vi "IACtrl_v2.vi"(7 "Irrigate?":bool=TRUE, 8 "Max Limit [mmHg]":dbl, 9 "E-Stop Vacuum":bool=TRUE, 10 "Vacuum Force [mmHg]":dbl) -> (1 "Accurus ChB Vout":dbl, 2 "Accurus ChA Vout":dbl, 3 "Accurus Engaged Vout":dbl, 6 "Vac Disp [mmHg]":i32)   [LabVIEW 2016]
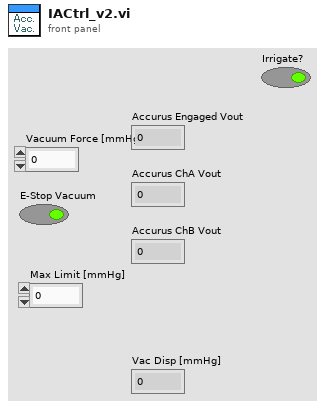
[diagram p1: front panel]
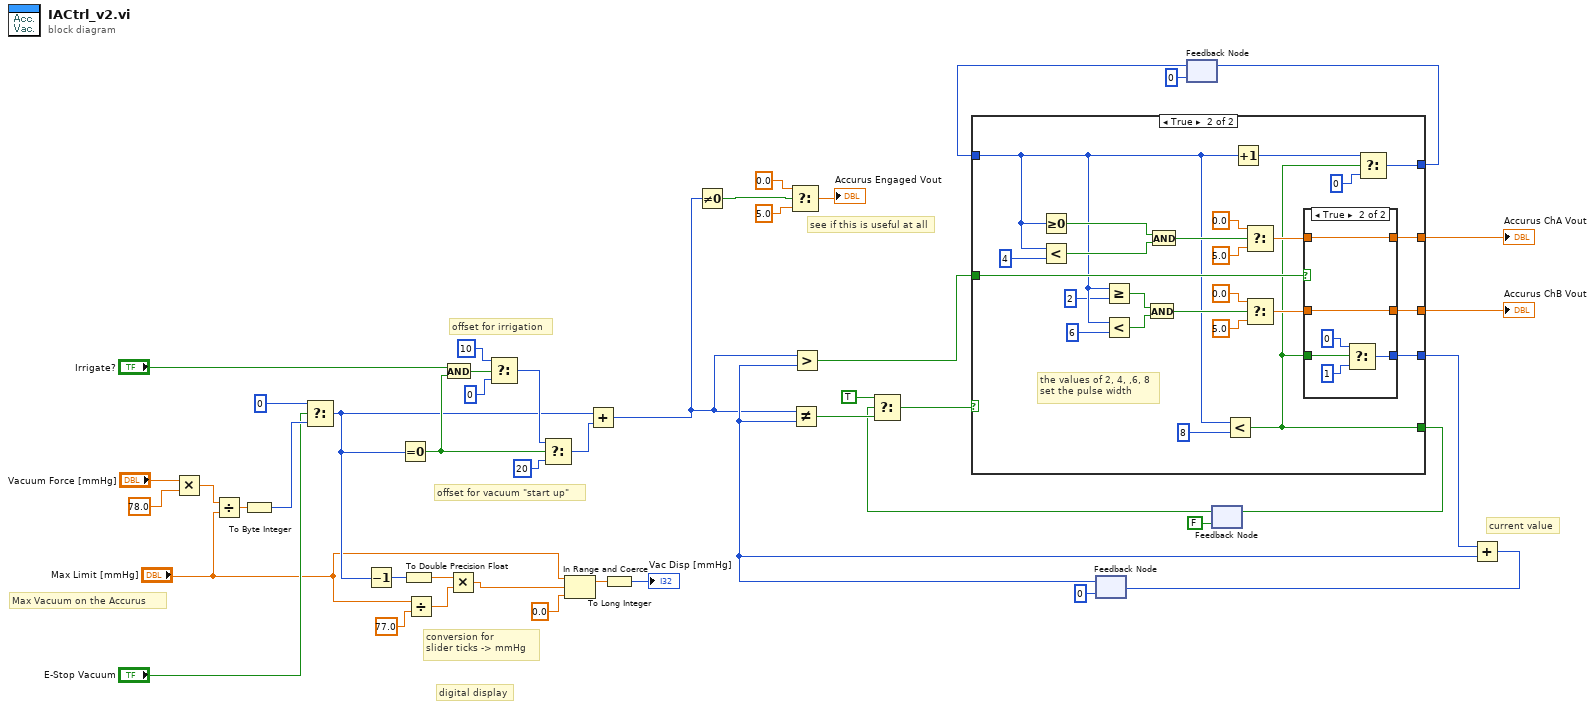
[diagram p0: block diagram]
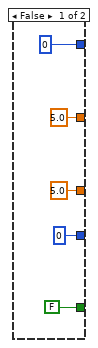
[diagram p2: hidden frame]
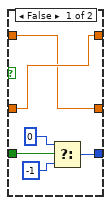
[diagram p3: hidden frame]
diagram:
  # "see if this is useful at all"
  # "digital display"
  # "offset for irrigation"
  # "Max Vacuum on the Accurus"
  # "conversion for\nslider ticks -> mmHg"
  # "offset for vacuum \"start up\""
  # "current value"
  n1 = Multiply(x="Vacuum Force [mmHg]", y=78.0) -> (x*y=w2:dbl)
  n2 = Divide(x=w2, y="Max Limit [mmHg]") -> (x/y=w16:dbl)
  n3 = To Byte Integer(number=w16) -> (8bit integer=w8:i8)
  n4 = Select(t=i8 0, s="E-Stop Vacuum", f=w8) -> (s? t:f=w7:i8)
  n5 = Decrement(x=w7) -> (x-1=w20:i8)
  n6 = Equal To 0?(x=w7) -> (x = 0?=w15:bool)
  n7 = To Double Precision Float(number=w20) -> (double precision float=w46:dbl)
  n8 = Divide(x="Max Limit [mmHg]", y=77.0) -> (x/y=w18:dbl)
  n9 = And(x="Irrigate?", y=w15) -> (x .and. y?=w14:bool)
  n10 = Multiply(x=w46, y=w18) -> (x*y=w17:dbl)
  n11 = Select(t=i8 10, s=w14, f=i8 0 ("t")) -> (s? t:f=w10:i8)
  n12 = Select(t=w10, s=w15, f=i8 20) -> (s? t:f=w43:i8)
  n13 = In Range and Coerce(upper limit="Max Limit [mmHg]", x=w17, lower limit=0.0) -> (coerced(x)=w21:dbl)  [unwired: 1 out]
  n14 = Add(x=w7, y=w43) -> (x+y=w9:i8)
  n15 = To Long Integer(number=w21) -> (32bit integer=→"Vac Disp [mmHg]":i32)
  n16 = Not Equal To 0?(x=w9) -> (x != 0?=w11:bool)
  n17 = Select(t=0.0, s=w11, f=5.0) -> (s? t:f=→"Accurus Engaged Vout":dbl)
  n18 = feedback #1(i8 0) -> (w29:i8)
  n19 = Not Equal?(x=w9, y=w29) -> (x != y?=w35:bool)
  n20 = Greater?(x=w9, y=w29) -> (0:w25:bool)
  n21 = feedback #2(i8 0) -> (w31:i8)
  n22 = feedback #3(FALSE) -> (w32:bool)
  n23 = Select(t=TRUE, s=w32, f=w35) -> (s? t:f=w34:bool)
  n24 = case shown="True" w34 {
    tunnel: [5.0 ("f") w64] -> w39
    tunnel: [5.0 ("f") w63] -> w40
    tunnel: [i8 0 ("f") w61] -> w28
    tunnel: [FALSE w56] -> w24
    tunnel: w25 -> [_ w62]
    tunnel: [i8 0 w58] -> w26
    tunnel: w31 -> [_ w60]
    frame False {
    }
    frame True {
      # "the values of 2, 4, ,6, 8 \nset the pulse width"
      n25 = Greater Or Equal To 0?(x=w60) -> (x >= 0?=w71:bool)
      n26 = Less?(x=w60, y=i8 4) -> (x < y?=w70:bool)
      n27 = Greater Or Equal?(x=w60, y=i8 2) -> (x >= y?=w69:bool)
      n28 = Less?(x=w60, y=i8 6) -> (x < y?=w68:bool)
      n29 = And(x=w69, y=w68) -> (x .and. y?=w67:bool)
      n30 = And(x=w71, y=w70) -> (x .and. y?=w72:bool)
      n31 = Less?(x=w60, y=i8 8) -> (x < y?=w56:bool)
      n32 = Increment(x=w60) -> (x+1=w59:i8)
      n33 = Select(t=0.0, s=w72, f=5.0) -> (s? t:f=w66:dbl)
      n34 = Select(t=0.0, s=w67, f=5.0) -> (s? t:f=w65:dbl)
      n35 = case shown="True" w62 {
        tunnel: w66 -> [w81 w87]
        tunnel: w65 -> [w82 w88]
        tunnel: [w81 w88] -> w63
        tunnel: [w82 w87] -> w64
        tunnel: w56 -> [w77 w86]
        tunnel: [w78 w85] -> w61
        frame False {
          n36 = Select(t=i8 0, s=w77, f=i8 -1) -> (s? t:f=w78:i8)
        }
        frame True {
          n37 = Select(t=i8 0, s=w86, f=i8 1) -> (s? t:f=w85:i8)
        }
      }
      n38 = Select(t=w59, s=w56, f=i8 0) -> (s? t:f=w58:i8)
    }
  }
  "Accurus ChB Vout" <- w40
  "Accurus ChA Vout" <- w39
  n39 = feedback-in #2(w26) -> ()
  n40 = feedback-in #3(w24) -> ()
  n41 = Add(x=w28, y=w29) -> (x+y=w45:i8)
  n42 = feedback-in #1(w45) -> ()
